vi "convert_dat2tdms.vi"() -> ()   [LabVIEW 2010]
panel:
  out "New Filel Path":path
  in  "Path":path=path "C:/skil/78-2009_11_26-11_08_00.dat"
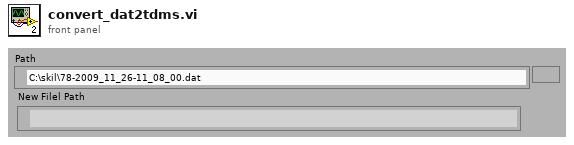
[diagram p1: front panel]
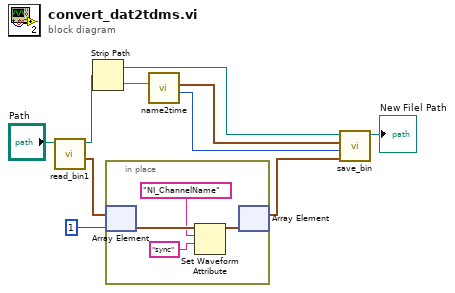
[diagram p0: block diagram]
diagram:
  n1 = call "read_bin1.vi"("Path"="Path") -> ("Waveform Graph"=w5:waveform(i16)[], "new file path"=w10:path)  [unwired: 4 in, 1 out]
  n2 = Strip Path(path=w10) -> (stripped path=w6:path, name=w9:string)
  n3 = in-place {
    n4 = in-place-array #1(w5, 1 ("index")) -> (w14:waveform(i16))
    n5 = Set Waveform Attribute(5:"sync", 6:"NI_ChannelName" ("name"), 7:w14) -> (3:w13:waveform(i16))  [unwired: 1 in, 2 out]
    n6 = in-place-array #1(w13) -> (w3:waveform(i16)[])  [unwired: 1 out]
  }
  n7 = call "name2time.vi"("f_name"=w9) -> ("m_pt"=w8:i32, "time stamp"=w7:timestamp)  [unwired: 4 in, 1 out]
  n8 = call "save_bin.vi"("SigArray"=w3, "DevNo"=w8, "timestamp"=w7, "start path"=w6) -> ("final Path"=→"New Filel Path":path)  [unwired: 2 in, 1 out]
